vi "Send Acyclic Frame.vi"(6 "Index":i32=1, 8 "error in (no error)":errorcluster, 9 "Device Reference in":T16 format="%.0x", 11 "RT Data out":T1 {"Acyclic Frame Refs" format="%.0x"; "Label Transfer Config"."Block Data Refs"."Data Reference" format="%.0x"; "Status Config"."HWOut Dur Ref" format="%.0x"; "Status Config"."HWIn Dur Ref" format="%.0x"; "Status Config"."HWOut Count Ref" format="%.0x"; "Status Config"."HWIn Count Ref" format="%.0x"; "Status Config"."Error Data Ref" format="%.0x"; "HWOutput Channels"."Message Settings"."Driver Data"."First Word" min=8 max=31; "HWOutput Channels"."Message Settings"."Driver Data"."Num Bits" min=1 max=32; "HWOutput Channels"."Message Settings"."Driver Data"."Start Bit" min=8 max=31; "HWOutput Channels"."Message Settings"."Block Data Refs"."Data Reference" format="%.0x"; "HWInput Channels"."Message Settings"."Driver Data"."First Word" min=8 max=31; "HWInput Channels"."Message Settings"."Driver Data"."Num Bits" min=1 max=32; "HWInput Channels"."Message Settings"."Driver Data"."Start Bit" min=8 max=31; "HWInput Channels"."Message Settings"."Block Data Refs"."Data Reference" format="%.0x"}) -> (0 "error out":errorcluster)   [LabVIEW 2013, in "AIT 1553 Custom Device.lvlib"]
uses:
  AIT 1553 Custom Device.lvlib
  <vilib>/NI Veristand/Custom Device API/Custom Device Item Ref.ctl
  RT Controls/AIT 1553  - RT Data.ctl
  RT Controls/AIT 1553 - RT HW Channel.ctl
  RT Controls/AIT 1553 - Bus Section.ctl
  RT Controls/AIT 1553 - RT Message Settings.ctl
  <vilib>/NI Veristand/Custom Device API/Block Data Reference.ctl
  <vilib>/NI Veristand/Custom Device API/Data Reference.ctl
  RT Controls/AIT 1553 - Driver Data.ctl
  Controls and Global/Start Bit.ctl
  Controls and Global/Number of Bits.ctl
  RT Controls/AIT 1553 - Board Config Info.ctl
  RT Controls/AIT 1553 - Hardware Type.ctl
  RT Controls/Error Qs.ctl
  RT Controls/Status Channels Config.ctl
  RT Controls/FIFO.ctl
  RT Controls/Label Transfer Config.ctl
  <vilib>/NI Veristand/Custom Device API/Data Access Type.ctl
  <vilib>/NI Veristand/Custom Device API/Global Data Refs.vi
  <vilib>/NI Veristand/Custom Device API/Custom Device API.lvlib
  <userlib>/MIL-STD-1553/Owl1553.lvlib
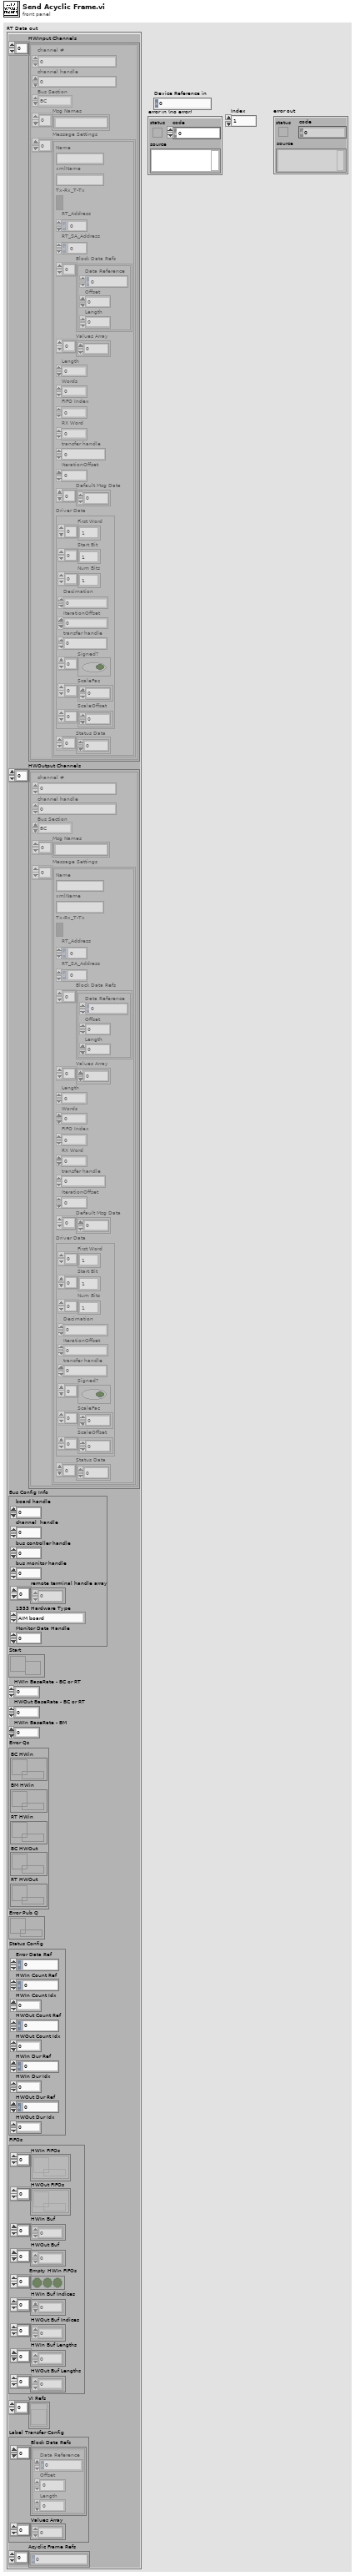
[diagram p1: front panel]
types:
  T1 = typedef "AIT 1553 Custom Device.lvlib/AIT 1553  - RT Data.ctl" = cluster{"HWInput Channels":T2[], "HWOutput Channels":T2[], "Bus Config Info":T10, "Start":refnum<notifier>, "HWIn BaseRate - BC or RT":i64, "HWOut BaseRate - BC or RT":i64, "HWIn BaseRate - BM":i64, "Error Qs":T12, "Error Pub Q":refnum<queue>, "Status Config":T13, "FIFOs":T14, "VI Refs":refnum<vi>[], "Label Transfer Config":T15, "Acyclic Frame Refs":T16[]}
  T2 = typedef "AIT 1553 Custom Device.lvlib/AIT 1553 - RT HW Channel.ctl" = cluster{"channel #":u16, "channel handle":u32, "Bus Section":T3, "Msg Names":string[], "Message Settings":T4[]}
  T3 = typedef "AIT 1553 Custom Device.lvlib/AIT 1553 - Bus Section.ctl" = enum16{"BC", "BM", "RT"}
  T4 = typedef "AIT 1553 Custom Device.lvlib/AIT 1553 - RT Message Settings.ctl" = cluster{"Name":string, "xmlName":string, "Tx-Rx_T-Tx":bool, "RT_Address":u8, "RT_SA_Address":u8, "Block Data Refs":T5[], "Values Array":dbl[], "Length":i32, "Words":i32, "FIFO Index":i32, "RX Word":u32, "transfer handle":u32, "IterationOffset":i32, "Default Msg Data":u16[], "Driver Data":T7, "Status Data":u32[]}
  T5 = typedef "Custom Device API.lvlib/Block Data Reference.ctl" = cluster{"Data Reference":T6, "Offset":i32, "Length":i32}
  T6 = typedef "Custom Device API.lvlib/Data Reference.ctl" = i32
  T7 = typedef "AIT 1553 Custom Device.lvlib/AIT 1553 - Driver Data.ctl" = cluster{"First Word":T8[], "Start Bit":T8[], "Num Bits":T9[], "Decimation":i32, "IterationOffset":i32, "transfer handle":u32, "Signed?":bool[], "ScaleFac":dbl[], "ScaleOffset":dbl[]}
  T8 = typedef "AIT 1553 Custom Device.lvlib/Start Bit.ctl" = i32
  T9 = typedef "AIT 1553 Custom Device.lvlib/Number of Bits.ctl" = i32
  T10 = typedef "AIT 1553 Custom Device.lvlib/AIT 1553 - Board Config Info.ctl" = cluster{"board handle":u32, "channel  handle":u32, "bus controller handle":u32, "bus monitor handle":u32, "remote terminal handle array":u32[], "1553 Hardware Type":T11, "Monitor Data Handle":u32}
  T11 = typedef "AIT 1553 Custom Device.lvlib/AIT 1553 - Hardware Type.ctl" = enum16{"AIM board", "AIT Board"}
  T12 = typedef "AIT 1553 Custom Device.lvlib/Error Qs.ctl" = cluster{"BC HWin":refnum<queue>, "BM HWin":refnum<queue>, "RT HWin":refnum<queue>, "BC HWOut":refnum<queue>, "RT HWOut":refnum<queue>}
  T13 = typedef "AIT 1553 Custom Device.lvlib/Status Channels Config.ctl" = cluster{"Error Data Ref":T6, "HWIn Count Ref":T6, "HWIn Count Idx":i32, "HWOut Count Ref":T6, "HWOut Count Idx":i32, "HWIn Dur Ref":T6, "HWIn Dur Idx":i32, "HWOut Dur Ref":T6, "HWOut Dur Idx":i32}
  T14 = typedef "AIT 1553 Custom Device.lvlib/FIFO.ctl" = cluster{"HWIn FIFOs":refnum<k33>[], "HWOut FIFOs":refnum<k33>[], "HWIn Buf":dbl[], "HWOut Buf":dbl[], "Empty HWIn FIFOs":bool[], "HWIn Buf Indices":i32[], "HWOut Buf Indices":i32[], "HWIn Buf Lengths":i32[], "HWOut Buf Lengths":i32[]}
  T15 = typedef "AIT 1553 Custom Device.lvlib/Label Transfer Config.ctl" = cluster{"Block Data Refs":T5[], "Values Array":dbl[]}
  T16 = typedef "Custom Device API.lvlib/Custom Device Item Ref.ctl" = u64
  T17 = typedef "Custom Device API.lvlib/Data Access Type.ctl" = enum16{"Read", "Write"}
  T18 = typedef "Custom Device API.lvlib/Custom Device Item Info.ctl" = cluster{"Name":string, "Is Channel":bool, "GUID":string, "Is Waveform":bool}
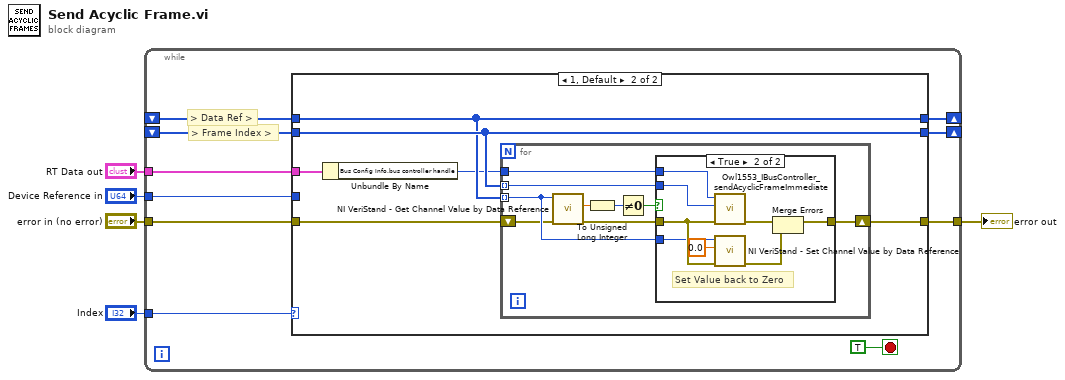
[diagram p0: block diagram]
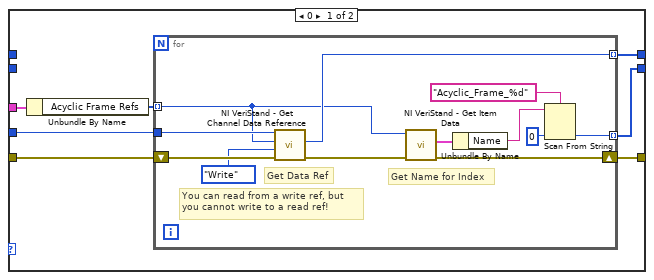
[diagram p2: hidden frame]
diagram:
  n1 = while {
    tunnel: "error in (no error)" -> [w15]
    tunnel: [w14] -> w4
    shift-right: [w12] -> _
    shift-left: _ -> [w11]
    tunnel: "Index" -> [w10]
    shift-right: [w7] -> _
    shift-left: _ -> [w8]
    tunnel: "Device Reference in" -> [w9]
    tunnel: "RT Data out" -> [w6]
    stop <- TRUE stop-if-true
    # "> Frame Index >"
    # "> Data Ref >"
    n2 = case shown="1, Default" w10 {
      tunnel: w15 -> [w22 w40]
      tunnel: [w21 w39] -> w14
      tunnel: [w16 w38] -> w12
      tunnel: w11 -> [_ w38]
      tunnel: w9 -> [w20 _]
      tunnel: w8 -> [_ w37]
      tunnel: [w19 w37] -> w7
      tunnel: w6 -> [w18 w36]
      frame 0 {
        n3 = Unbundle By Name(w18) -> ("Acyclic Frame Refs"=w17:T16[])
        n4 = for {
          tunnel: w17 -> [w24] mode=indexing
          shift-right: [w33] -> w21
          shift-left: w22 -> [w28]
          tunnel: [w30] -> w16 mode=indexing
          tunnel: w20 -> [w25]
          tunnel: [w26] -> w19 mode=indexing
          # "You can read from a write ref, but \nyou cannot write to a read ref!"
          # "Get Name for Index"
          # "Get Data Ref"
          n5 = call <vilib>:"NI VeriStand - Get Channel Data Reference.vi"("error in (no error)"=w28, "Access"=Data_Access_Type."Write", "Channel Ref in"=w24, "Device Ref in"=w25) -> ("error out"=w27:errorcluster, "Channel Data Reference"=w26:T6)  [unwired: 5 in, 1 out]
          n6 = call <vilib>:"NI VeriStand - Get Item Data.vi"("error in (no error)"=w27, "Item Ref in"=w24) -> ("error out"=w33:errorcluster, "Item Info"=w34:T18)  [unwired: 6 in, 2 out]
          n7 = Unbundle By Name(w34) -> ("Name"=w31:string)
          n8 = Scan From String(format string="Acyclic_Frame_%d", input string=w31, default 1=u32 0 ("acyclic index")) -> (output 1=w30:u32)  [unwired: 2 in, 3 out]
        }
      }
      frame 1, Default {
        n9 = Unbundle By Name(w36) -> ("Bus Config Info.bus controller handle"=w35:u32)
        n10 = for {
          shift-right: [w45] -> w39
          shift-left: w40 -> [w41]
          tunnel: w35 -> [w44]
          tunnel: w38 -> [w43] mode=indexing
          tunnel: w37 -> [w42] mode=indexing
          n11 = call <vilib>:"NI VeriStand - Get Channel Value by Data Reference.vi"("error in (no error)"=w41, "Data Reference in"=w42) -> ("error out"=w46:errorcluster, "Value"=w49:dbl)  [unwired: 8 in]
          n12 = To Unsigned Long Integer(number=w49) -> (unsigned 32bit integer=w48:u32)
          n13 = Not Equal To 0?(x=w48) -> (x != 0?=w47:bool)
          n14 = case shown="True" w47 {
            tunnel: w46 -> [w50 w58]
            tunnel: w42 -> [_ w57]
            tunnel: [w50 w53] -> w45
            tunnel: w44 -> [_ w52]
            tunnel: w43 -> [_ w51]
            frame False {
            }
            frame True {
              # "Set Value back to Zero"
              n15 = call <userlib>:"Owl1553_IBusController_sendAcyclicFrameImmediate.vi"("error in (no error)"=w58, "acyclic index"=w51, "bus controller handle"=w52) -> ("error out"=w55:errorcluster)  [unwired: 7 in, 1 out]
              n16 = call <vilib>:"NI VeriStand - Set Channel Value by Data Reference.vi"("error in (no error)"=w58, "Value"=0.0, "Data Reference in"=w57) -> ("error out"=w54:errorcluster)  [unwired: 8 in]
              n17 = Merge Errors(w55, w54) -> (w53:errorcluster)
            }
          }
        }
      }
    }
  }
  "error out" <- w4
